vi "Page_Advanced_ReadAll.vi"(6 "ctl references":T1, 8 "error in (no error)":errorcluster, 10 "Calculated IncludeHWConfig":bool, 11 "AB_Application in":refnum<class "AB_Application.lvclass">) -> (0 "error out":errorcluster, 3 "AB_Application out":refnum<class "AB_Application.lvclass">)   [LabVIEW 2020, in "AB_Application.lvclass"]
uses:
  <vilib>/AppBuilder/AB_Classes/Application/AB_Application.lvclass
  <vilib>/AppBuilder/AB_Classes/Application/AB_Application.lvclass/AB_Application.ctl
  <vilib>/AppBuilder/AB_Classes/TargetFile/AB_Targetfile.lvclass
  e:/builds/penguin/labview/branches/2020/dev/dist/vi.lib/AppBuilder/AB_Classes/TargetFile/AB_Targetfile.lvclass
  e:/builds/penguin/labview/branches/2020/dev/dist/vi.lib/AppBuilder/AB_Classes/Build/AB_Build.lvclass
  e:/builds/penguin/labview/branches/2020/dev/dist/vi.lib/AppBuilder/AB_Classes/Application/AB_Application.lvclass
  <resource>/Framework/Providers/Builds/AppBuilder/AB_UI_Page_Advanced_References.ctl
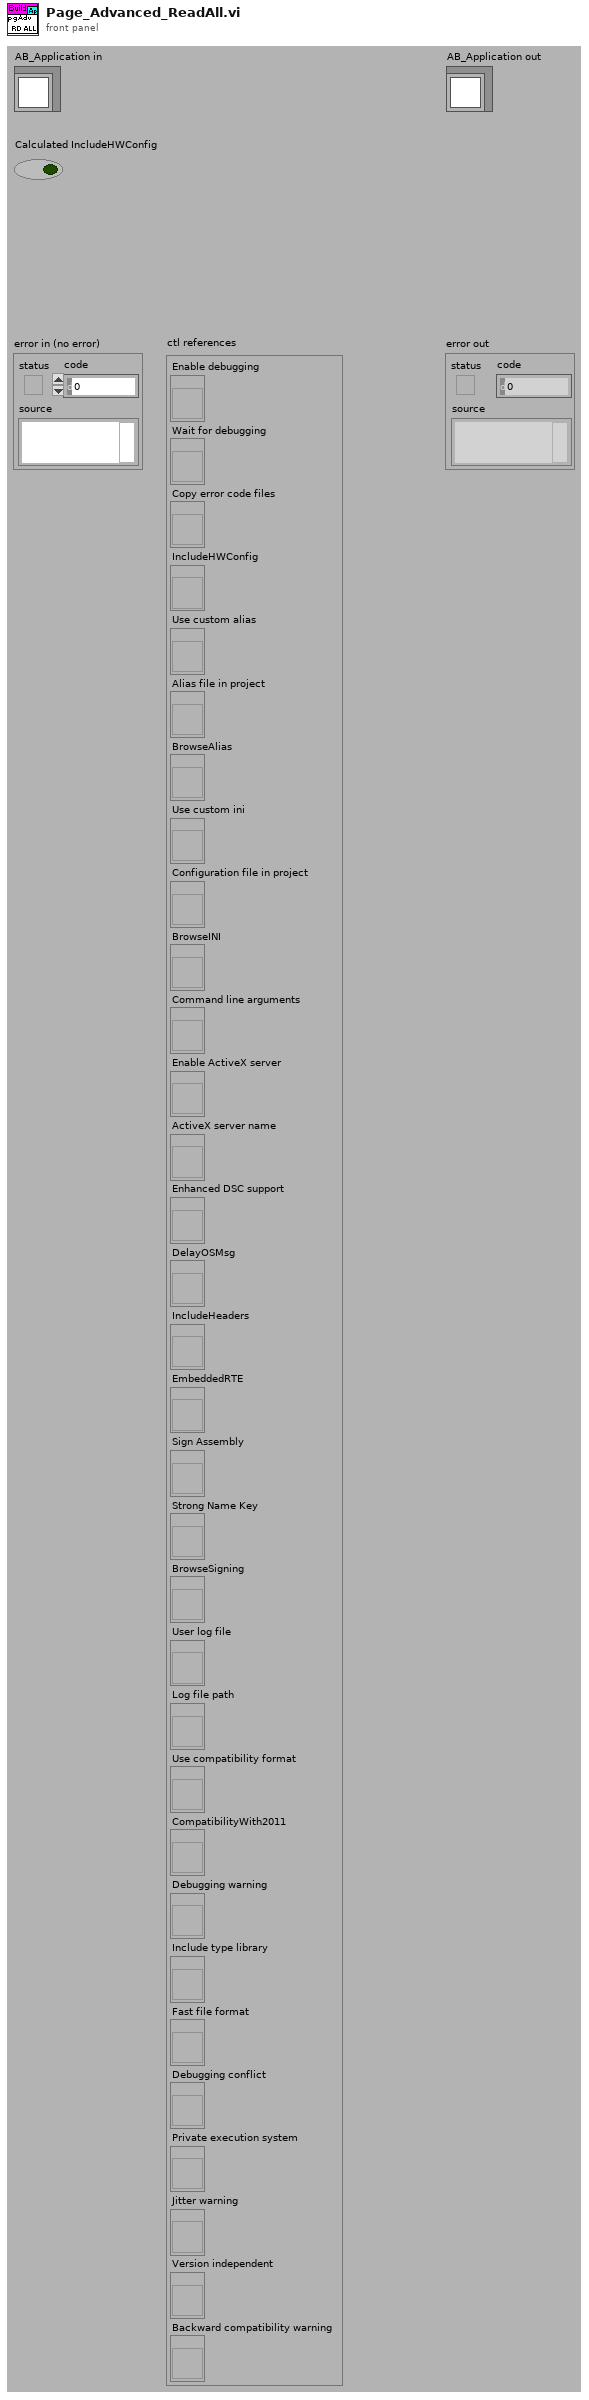
[diagram p1: front panel]
types:
  T1 = typedef "AB_UI_Page_Advanced_References.ctl" = cluster{"Enable debugging":refnum<vi>, "Wait for debugging":refnum<vi>, "Copy error code files":refnum<vi>, "IncludeHWConfig":refnum<vi>, "Use custom alias":refnum<vi>, "Alias file in project":refnum<vi>, "BrowseAlias":refnum<vi>, "Use custom ini":refnum<vi>, "Configuration file in project":refnum<vi>, "BrowseINI":refnum<vi>, "Command line arguments":refnum<vi>, "Enable ActiveX server":refnum<vi>, "ActiveX server name":refnum<vi>, "Enhanced DSC support":refnum<vi>, "DelayOSMsg":refnum<vi>, "IncludeHeaders":refnum<vi>, "EmbeddedRTE":refnum<vi>, "Sign Assembly":refnum<vi>, "Strong Name Key":refnum<vi>, "BrowseSigning":refnum<vi>, "User log file":refnum<vi>, "Log file path":refnum<vi>, "Use compatibility format":refnum<vi>, "CompatibilityWith2011":refnum<vi>, "Debugging warning":refnum<vi>, "Include type library":refnum<vi>, "Fast file format":refnum<vi>, "Debugging conflict":refnum<vi>, "Private execution system":refnum<vi>, "Jitter warning":refnum<vi>, "Version independent":refnum<vi>, "Backward compatibility warning":refnum<vi>}
  T2 = enum8{"Enabled", "Disabled", "Disabled and Grayed Out"}
  T3 = typedef "AB_Targetfile.ctl" = cluster{"targetfileName":string, "targetfileGUID":string, "enableDebugging":bool, "versionInfo":cluster{"productName":string, "legalCopyright":string, "companyName":string, "internalName":string, "fileDescription":string}, "eng_consolidatedTypeInfo":string, "fastFileFormat":bool, "eng_LEIFBuildData":u32, "versionIndependent":bool}
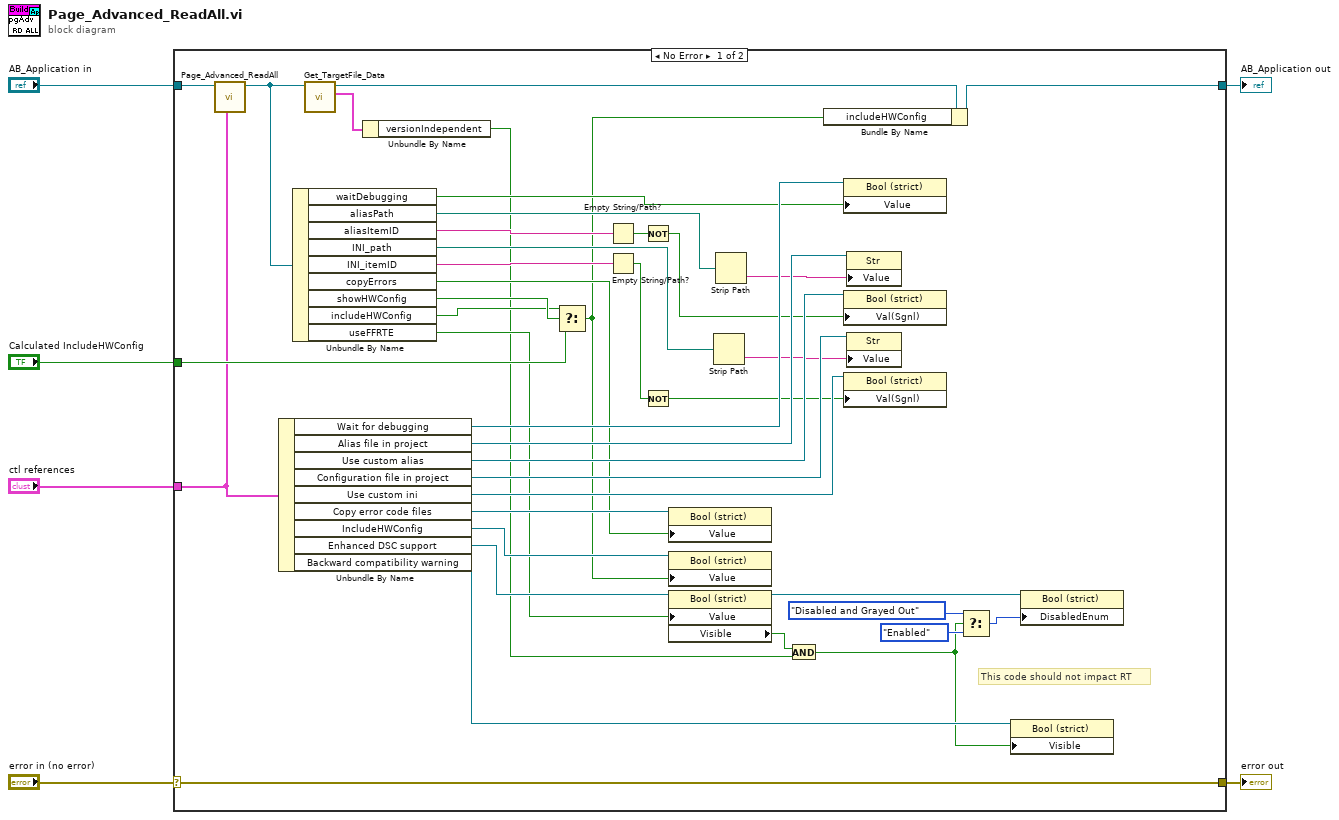
[diagram p0: block diagram]
diagram:
  n1 = case shown="No Error" "error in (no error)" {
    selector: "error in (no error)" -> [w11 w48]
    tunnel: [w11 w48] -> w5
    tunnel: [w46 w47] -> w3
    tunnel: "AB_Application in" -> [w23 w47]
    tunnel: "ctl references" -> [w22 _]
    tunnel: "Calculated IncludeHWConfig" -> [w25 _]
    frame No Error {
      # "This code should not impact RT"
      n2 = call-parent "Page_Advanced_ReadAll.vi"("ctl references"=w22, "AB_Targetfile in"=w23) -> ("AB_Targetfile out"=w10:refnum<class "AB_Application.lvclass">)  [unwired: 2 in, 7 out]
      n3 = Unbundle By Name(w22) -> ("Wait for debugging"=w45:refnum<vi>, "Alias file in project"=w42:refnum<vi>, "Use custom alias"=w39:refnum<vi>, "Configuration file in project"=w36:refnum<vi>, "Use custom ini"=w34:refnum<vi>, "Copy error code files"=w31:refnum<vi>, "IncludeHWConfig"=w30:refnum<vi>, "Enhanced DSC support"=w29:refnum<vi>, "Backward compatibility warning"=w19:refnum<vi>)
      n4 = Unbundle By Name(w10) -> ("waitDebugging"=w44:bool, "aliasPath"=w43:path, "aliasItemID"=w40:string, "INI_path"=w37:path, "INI_itemID"=w33:string, "copyErrors"=w28:bool, "showHWConfig"=w27:bool, "includeHWConfig"=w26:bool, "useFFRTE"=w18:bool)
      n5 = call <vilib>:"Get_TargetFile_Data.vi"("AB_Targetfile in"=w10) -> ("data"=w8:T3, "AB_Targetfile out"=w9:refnum<class "AB_Application.lvclass">)  [unwired: 8 in, 1 out]
      n6 = Unbundle By Name(w8) -> ("versionIndependent"=w7:bool)
      n7 = Select(t=w26, s=w27, f=w25) -> (s? t:f=w24:bool)
      n8 = Empty String/Path?(string/path=w40) -> (empty?=w38:bool)
      n9 = Empty String/Path?(string/path=w33) -> (empty?=w32:bool)
      n10 = Not(x=w38) -> (.not. x?=w21:bool)
      n11 = Not(x=w32) -> (.not. x?=w20:bool)
      n12 = property class="Bool (strict)"(reference=w31, "Value"=w28) -> ()  [unwired: 1 in, 2 out]
      n13 = property class="Bool (strict)"(reference=w30, "Value"=w24) -> ()  [unwired: 1 in, 2 out]
      n14 = property class="Bool (strict)"(reference=w29, "Value"=w18) -> (reference out=w14:refnum<vi>, "Visible"=w15:bool)  [unwired: 1 in, 1 out]
      n15 = Strip Path(path=w37) -> (name=w35:string)  [unwired: 1 out]
      n16 = Strip Path(path=w43) -> (name=w41:string)  [unwired: 1 out]
      n17 = And(x=w15, y=w7) -> (x .and. y?=w12:bool)
      n18 = Bundle By Name(cluster=w9, "includeHWConfig"=w24) -> (w46:refnum<class "AB_Application.lvclass">)
      n19 = property class="Bool (strict)"(reference=w45, "Value"=w44) -> ()  [unwired: 1 in, 2 out]
      n20 = property class="Bool (strict)"(reference=w39, "Val(Sgnl)"=w21) -> ()  [unwired: 1 in, 2 out]
      n21 = property class="Bool (strict)"(reference=w34, "Val(Sgnl)"=w20) -> ()  [unwired: 1 in, 2 out]
      n22 = property class="Str"(reference=w42, "Value"=w41) -> ()  [unwired: 1 in, 2 out]
      n23 = property class="Str"(reference=w36, "Value"=w35) -> ()  [unwired: 1 in, 2 out]
      n24 = Select(t=T2."Disabled and Grayed Out" ("Disabled"), s=w12, f=T2."Enabled" ("Disabled")) -> (s? t:f=w13:T2)
      n25 = property class="Bool (strict)"(reference=w19, "Visible"=w12) -> ()  [unwired: 1 in, 2 out]
      n26 = property class="Bool (strict)"(reference=w14, "DisabledEnum"=w13) -> ()  [unwired: 1 in, 2 out]
    }
    frame Error {
    }
  }
  "error out" <- w5
  "AB_Application out" <- w3
